vi "ATF-Pump-Digital input build to analog.vi"(7 "Samples":i32=10, 10 "DI":digitalwaveform[](array[waveform]), 11 "RD.AI_C_Data RD":refnum<queue>) -> ()   [LabVIEW 2022 SP3]
uses:
  <vilib>/Waveform/DTblOps.llb/DTbl Digital to Boolean Array.vi
panel:
  in  "DI_Data RD":refnum<queue>
  out "overflow?":bool
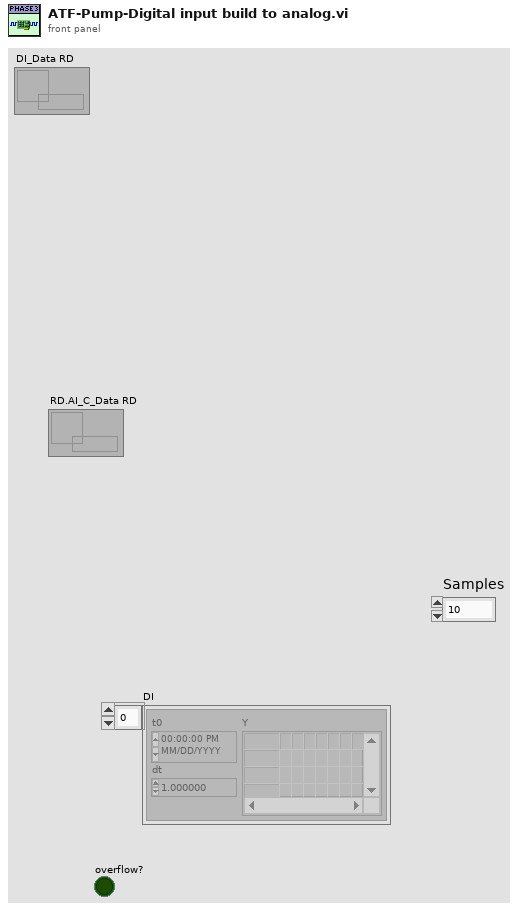
[diagram p1: front panel]
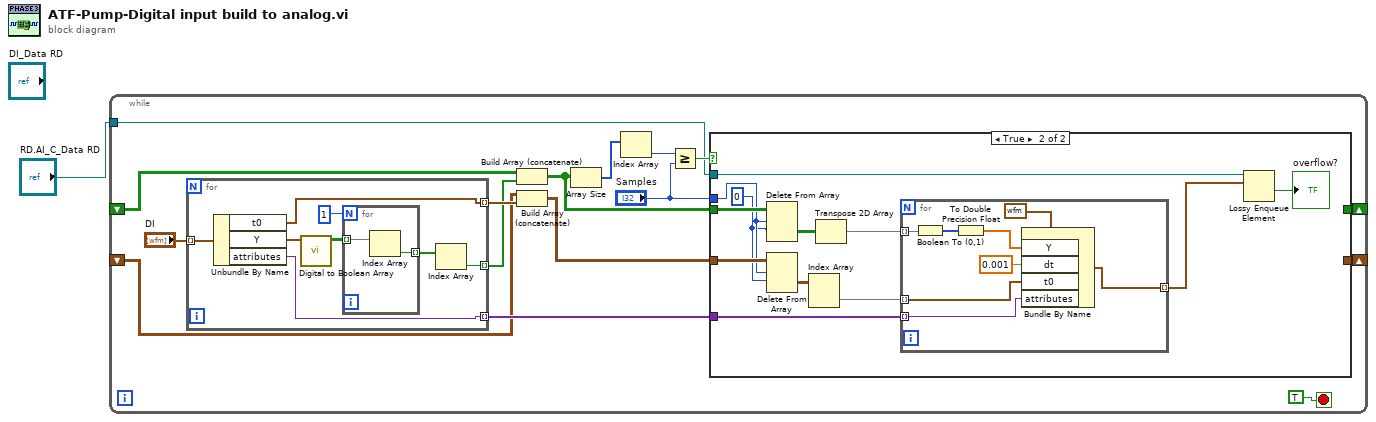
[diagram p0: block diagram]
diagram:
  n1 = while {
    shift-right: [w5] -> _
    shift-left: _ -> [w6]
    shift-right: [w4] -> _
    shift-left: _ -> [w7]
    tunnel: "RD.AI_C_Data RD" -> [w2]
    stop <- TRUE stop-if-true
    n2 = for {
      tunnel: "DI" -> [w47] mode=indexing
      tunnel: [w40] -> w10 mode=indexing
      tunnel: [w46] -> w15 mode=indexing
      tunnel: [w45] -> w17 mode=indexing
      n3 = Unbundle By Name(w47) -> ("t0"=w46:timestamp, "Y"=w41:digitaldata, "attributes"=w45:variant)
      n4 = call-poly <vilib>:"Digital to Boolean Array.vi"("digital data"=w41) -> ("boolean array"=w43:bool[][])  [unwired: 9 in, 1 out]
      n5 = for {
        N: 1 -> [_]
        tunnel: w43 -> [w49] mode=indexing
        tunnel: [w48] -> w42 mode=indexing
        n6 = Index Array(array=w49) -> (element=w48:bool)  [unwired: 1 in]
      }
      n7 = Index Array(array=w42) -> (element=w40:bool)  [unwired: 1 in]
    }
    n8 = Build Array (concatenate)(w7, w10) -> (w13:bool[][])
    n9 = Build Array (concatenate)(w6, w15) -> (w16:timestamp[][])
    n10 = Array Size(array=w13) -> (size(s)=w11:i32[])
    n11 = Index Array(array=w11) -> (element=w12:i32)  [unwired: 1 in]
    n12 = Greater Or Equal?(x=w12, y="Samples") -> (x >= y?=w14:bool)
    n13 = case shown="True" w14 {
      tunnel: w13 -> [w19 w31]
      tunnel: [w19 _] -> w4
      tunnel: w16 -> [w18 w30]
      tunnel: [w18 _] -> w5
      tunnel: w17 -> [_ w27]
      tunnel: "Samples" -> [_ w26]
      tunnel: w2 -> [_ w24]
      frame False {
      }
      frame True {
        w21 = 0 ("index (row)")
        n14 = Delete From Array(array=w31, length=w26, index (row)=w21) -> (deleted portion=w23:bool[][])  [unwired: 1 in, 1 out]
        n15 = Delete From Array(array=w30, length=w26, index (row)=w21) -> (deleted portion=w29:timestamp[][])  [unwired: 1 in, 1 out]
        n16 = Index Array(array=w29) -> (element=w28:timestamp[])  [unwired: 2 in]
        n17 = Transpose 2D Array(2D array=w23) -> (transposed array=w22:bool[][])
        n18 = for {
          tunnel: w28 -> [w35] mode=indexing
          tunnel: w27 -> [w34] mode=indexing
          tunnel: w22 -> [w39] mode=indexing
          tunnel: [w32] -> w20 mode=indexing
          n19 = Boolean To (0,1)(Boolean=w39) -> (0, 1=w38:i16[])
          n20 = To Double Precision Float(number=w38) -> (double precision float=w37:dbl[])
          n21 = Bundle By Name(cluster=waveform(dbl) {"t0"=timestamp(0 s since 1904-01-01), "dt"=1.0, "Y"=[]} ("waveform"), "Y"=w37, "dt"=0.001, "t0"=w35, "attributes"=w34) -> (w32:waveform(dbl))
        }
        n22 = Lossy Enqueue Element(queue=w24, element=w20) -> (overflow?=→"overflow?":bool)  [unwired: 1 in, 3 out]
      }
    }
  }
